vi "File Write Orbit.vi"(7 "error in (no error)":errorcluster, 8 "BPM Reading Names":string[](array[string]), 9 "Orbit":dbl[](array[numeric]), 10 "file path (dialog if empty)":path) -> (0 "error out":errorcluster)   [LabVIEW 2011, in "File VIs.lvlib"]
doc: "Reads a numeric text file and converts the data to a 2D, double-precision array of numbers."
uses:
  File VIs.lvlib
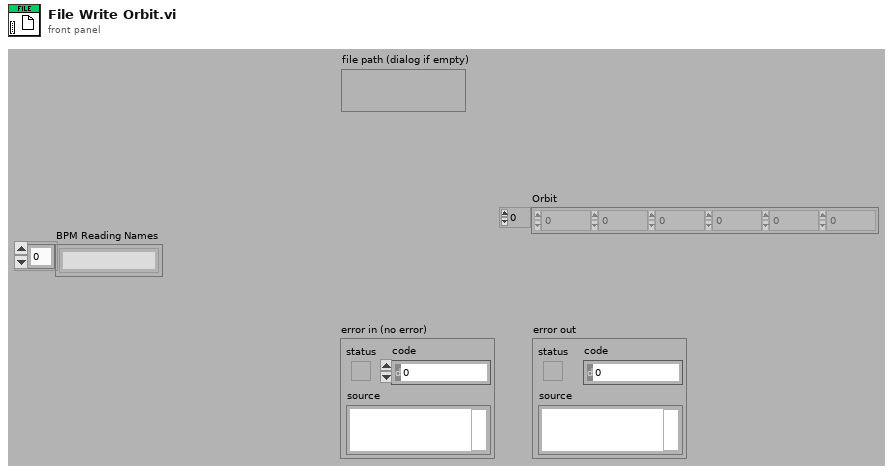
[diagram p1: front panel]
types:
  T1 = enum16{"open", "replace", "create", "open or create", "replace or create", "replace or create with confirmation"}
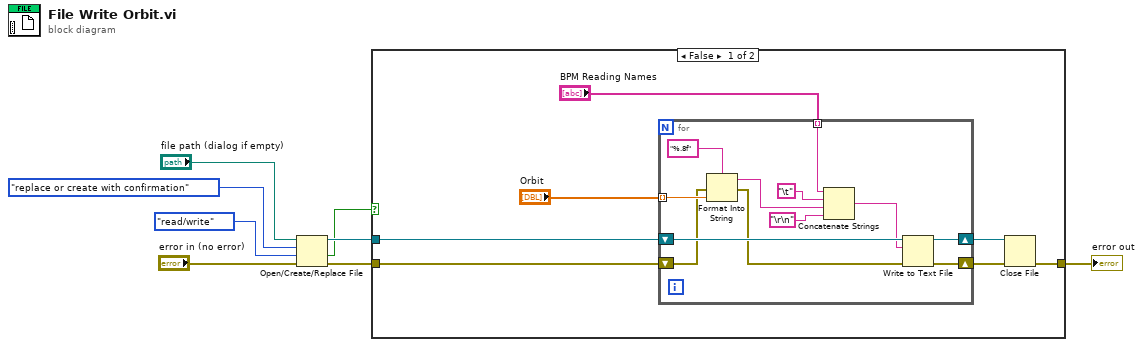
[diagram p0: block diagram]
diagram:
  n1 = Open/Create/Replace File(file path (use dialog)="file path (dialog if empty)", error in="error in (no error)", operation (0:open)=T1."replace or create with confirmation", access (0:read/write)=enum16{"read/write", "read-only", "write-only"}."read/write") -> (refnum out=w7:refnum<file>, cancelled=w1:bool, error out=w6:errorcluster)  [unwired: 2 in]
  n2 = case shown="False" w1 {
    tunnel: [w13 w28] -> w8
    tunnel: w7 -> [w12 _]
    tunnel: w6 -> [w11 w28]
    frame False {
      n3 = for {
        shift-right: [w26] -> w14
        shift-left: w11 -> [w19]
        shift-right: [w27] -> w15
        shift-left: w12 -> [w25]
        tunnel: "BPM Reading Names" -> [w24] mode=indexing
        tunnel: "Orbit" -> [w21] mode=indexing
        n4 = Format Into String(format string="%.8f", error in=w19, w21) -> (resulting string=w20:string, error out=w18:errorcluster)  [unwired: 1 in]
        n5 = Concatenate Strings(w24, "\t", w20, "\r\n") -> (w22:string)
        n6 = Write to Text File(file (use dialog)=w25, text=w22, error in=w18) -> (refnum out=w27:refnum<file>, error out=w26:errorcluster)  [unwired: 1 in, 1 out]
      }
      n7 = Close File(refnum=w15, error in=w14) -> (error out=w13:errorcluster)  [unwired: 1 out]
    }
    frame True {
    }
  }
  "error out" <- w8
